vi "StatusBits.vi"(10 "StatusBit":enum16{"LastSubsite", "LastDie"}(ring)) -> (2 "StatusBits":i32)   [LabVIEW 2015]
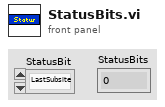
[diagram p1: front panel]
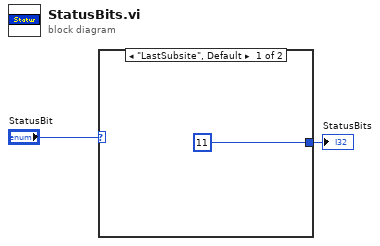
[diagram p0: block diagram]
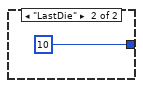
[diagram p2: hidden frame]
diagram:
  n1 = case shown="\"LastSubsite\", Default" "StatusBit" {
    tunnel: [11 10] -> w1
    frame "LastSubsite", Default {
    }
    frame "LastDie" {
    }
  }
  "StatusBits" <- w1
